vi "get channels removed since last load.vi"(11 "fixed channel configuration in":refnum<class "control module configuration.lvclass">) -> (2 "removed":refnum<class "TBM channel.lvclass">[](array[class]), 3 "fixed channel configuration out":refnum<class "control module configuration.lvclass">)   [LabVIEW 2013, in "control module configuration.lvclass"]
uses:
  control module configuration.lvclass
  <vilib>/NI/Tag Bus Module Framework/channel/TBM channel.lvclass
  control module configuration.lvclass/control module configuration.ctl
  <vilib>/NI/Tag Bus/tag/tag descriptor.lvclass/tag descriptor.ctl
  <vilib>/NI/Tag Bus Module Framework/channel/TBM channel.lvclass/TBM channel.ctl
  <vilib>/NI/Tag Bus/tag/read data type.vi
  <vilib>/NI/Tag Bus Module Framework/channel/Read channel classification.vi
  <vilib>/NI/Tag Bus/tag/read tag name.vi
  <vilib>/NI/Tag Bus/tag/tag descriptor.lvclass
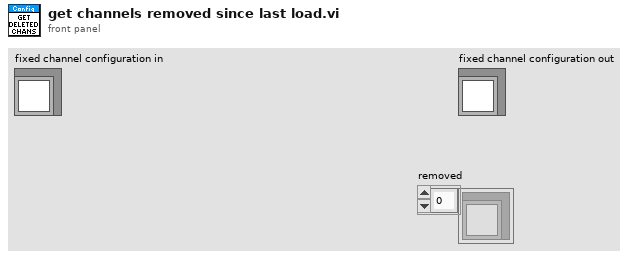
[diagram p1: front panel]
types:
  T1 = typedef "tag bus.lvlib/tag descriptor.lvclass/Data Type.ctl" = enum16{"Double", "Single", "I64", "I32", "I16", "I8", "U64", "U32", "U16", "U8", "Boolean", "String", "Array of Double", "Array of Single", "Array of I64", "Array of I32", "Array of I16", "Array of I8", "Array of U64", "Array of U32", "Array of U16", "Array of U8", "Array of Boolean", "Array of String"}
  T2 = typedef "TBM channel.lvclass/channel classification.ctl" = enum16{"input data", "output data", "processing parameter", "processing result"}
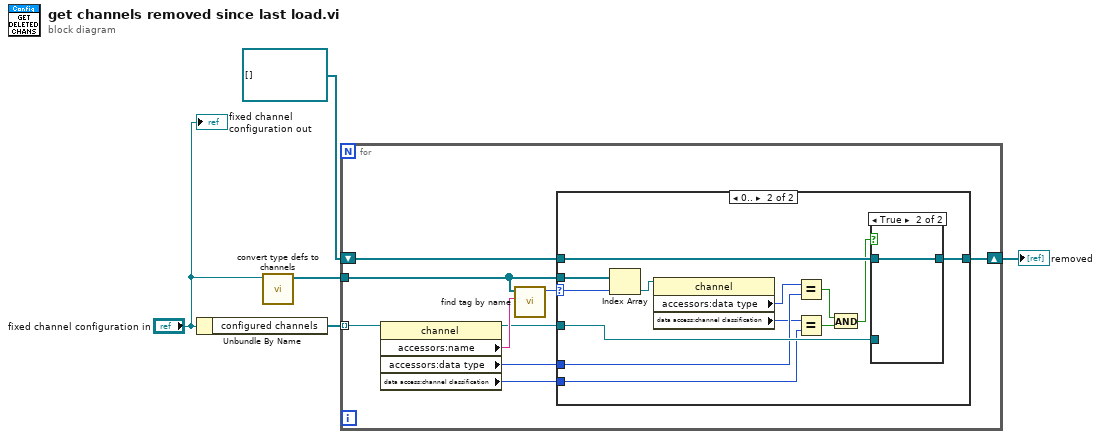
[diagram p0: block diagram]
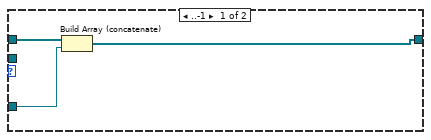
[diagram p2: hidden frame]
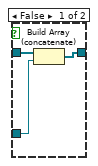
[diagram p3: hidden frame]
diagram:
  n1 = Unbundle By Name("fixed channel configuration in") -> ("configured channels"=w4:refnum<class "TBM channel.lvclass">[])
  n2 = call "convert type defs to channels.vi"("fixed channel configuration"="fixed channel configuration in") -> ("Array out"=w5:refnum<class "TBM channel.lvclass">[])  [unwired: 9 in, 1 out]
  n3 = for {
    tunnel: w4 -> [w14] mode=indexing
    shift-right: [w8] -> w1
    shift-left: refnum<class "TBM channel.lvclass">[] [] ("Array out") -> [w9]
    tunnel: w5 -> [w7]
    n4 = property class="channel"(reference=w14) -> (reference out=w10:refnum<class "TBM channel.lvclass">, "accessors:name"=w13:string, "accessors:data type"=w11:T1, "data access:channel classification"=w6:T2)  [unwired: 1 in, 1 out]
    n5 = call <vilib>:"find tag by name.vi"("name"=w13, "tags in"=w7) -> ("index"=w12:i32)  [unwired: 9 in]
    n6 = case shown="0.." w12 {
      selector: w12 -> [_ w29]
      tunnel: w11 -> [_ w23]
      tunnel: w10 -> [w16 w25]
      tunnel: w9 -> [w17 w27]
      tunnel: [w15 w26] -> w8
      tunnel: w7 -> [_ w30]
      tunnel: w6 -> [_ w18]
      frame ..-1 {
        n7 = Build Array (concatenate)(w17, w16) -> (w15:refnum<class "TBM channel.lvclass">[])
      }
      frame 0.. {
        n8 = Index Array(array=w30, index=w29) -> (element=w28:refnum<class "TBM channel.lvclass">)
        n9 = property class="channel"(reference=w28) -> ("accessors:data type"=w24:T1, "data access:channel classification"=w20:T2)  [unwired: 1 in, 2 out]
        n10 = Equal?(x=w24, y=w23) -> (x = y?=w21:bool)
        n11 = Equal?(x=w20, y=w18) -> (x = y?=w19:bool)
        n12 = And(x=w21, y=w19) -> (x .and. y?=w22:bool)
        n13 = case shown="True" w22 {
          tunnel: w27 -> [w33 w34]
          tunnel: [w32 w34] -> w26
          tunnel: w25 -> [w31 _]
          frame False {
            n14 = Build Array (concatenate)(w33, w31) -> (w32:refnum<class "TBM channel.lvclass">[])
          }
          frame True {
          }
        }
      }
    }
  }
  "removed" <- w1
  "fixed channel configuration out" <- "fixed channel configuration in"
